vi "Unflatten.vi"(7 "Release Lock":bool=TRUE, 8 "error in (no error)":errorcluster, 9 "Timeout":bool, 10 "DAQ In":T1[](array[typedef]), 11 "CIF_NIChn_FIFO_DAQ in":refnum<class "CIF_NIChn_FIFO_DAQ_DVR.lvclass">) -> (0 "error out":errorcluster, 1 "Header":T2, 2 "DAQ Out":T1[](array[typedef]), 3 "CIF_NIChn_FIFO_DAQ out":refnum<class "CIF_NIChn_FIFO_DAQ_DVR.lvclass">)   [LabVIEW 2021, in "CIF_NIChn_FIFO_DAQ_DVR.lvclass"]
uses:
  CIF_NIChn_FIFO_DAQ_DVR.lvclass
  D:/dev/Packages/Channel_Manager/src/CIFChannels/CIFChannels.lvclass
  D:/dev/Packages/Channel_Manager/src/CIF_NIChn/FIFO_U8/CIF_NIChn_Fifo_U8.lvclass
  ChannelCommon/typedef/FIFO Header.ctl
  ChannelCommon/typedef/Datatype Waveform.ctl
  CIFChannels/CIFChannels.lvclass/CIFChannels.ctl
  FIFO_U8/CIF_NIChn_Fifo_U8.lvclass/CIF_NIChn_Fifo_U8.ctl
  CIF_NIChn_FIFO_DAQ_DVR.lvclass/CIF_NIChn_FIFO_DAQ_DVR.ctl
  <vilib>/CIF Foundation/CIF Utilities/Statistics/I64/Stats_I64_CIF_U.lvclass/Stats_I64_CIF_U.ctl
  4ab41953-a001-49d2-beab-55370b6c3c42.vi
  7cd889b7-face-4678-a9e3-2692853b6930.vi
  CIFChannels/Accessors/Write FIFO Header.vi
  CIFChannels/Accessors/Write FIFO Timeout.vi
  FIFO_U8/Accessors/Read Payload.vi
  ChannelCommon/Utilities/Unflatten Header.vi
  ChannelCommon/Utilities/Add Error.vi
  <vilib>/CIF Foundation/CIF Utilities/DataTypes/Unflatten U64.vi
  <vilib>/CIF Foundation/CIF Utilities/Time/System Time/Get System Time.vi
  <vilib>/CIF Foundation/CIF Utilities/Statistics/I64/X1 minus X0.vi
  <vilib>/CIF Foundation/CIF Utilities/DataTypes/Unflatten I64.vi
  <vilib>/CIF Foundation/CIF Utilities/Errors/Append Error Location.vi
  <vilib>/CIF Foundation/CIF Utilities/Time/System Time/LabVIEW Time to TAI Time.vi
  <vilib>/CIF Foundation/CIF Utilities/Statistics/I64/X1 minus X0.vi/dfabcf33-0dbc-4041-80a5-3dc0c86d2989.vi
  <vilib>/CIF Foundation/CIF Utilities/Statistics/I64/X1 minus X0.vi/dfabcf33-0dbc-4041-80a5-3dc0c86d2989.vi/9eb60a9a-770f-4d2d-8b3f-8465c267ecc9.vi
  ChannelCommon/ChannelCommon.lvlib
  CIFChannels/CIFChannels.lvclass
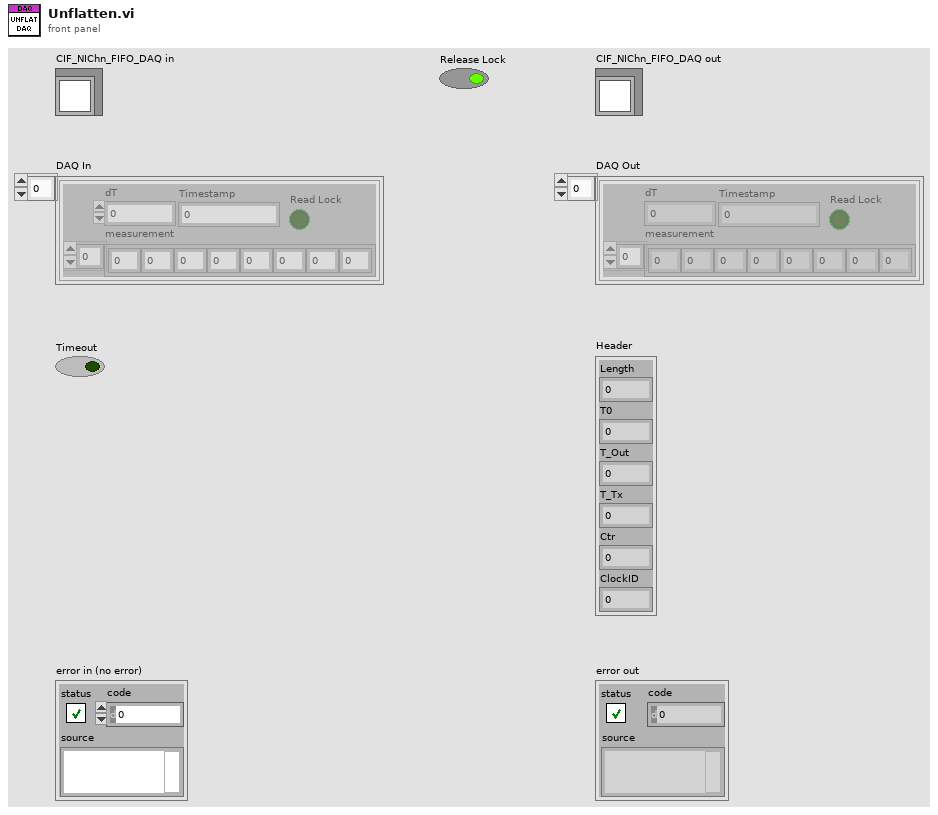
[diagram p1: front panel]
types:
  T1 = typedef "ChannelCommon.lvlib/Datatype Waveform.ctl" = cluster{"measurement":dbl[], "dT":dbl, "Timestamp":i64, "Read Lock":bool}
  T2 = typedef "ChannelCommon.lvlib/FIFO Header.ctl" = cluster{"Length":u64, "T0":i64, "T_Out":i64, "T_Tx":i64, "Ctr":u64, "ClockID":u8}
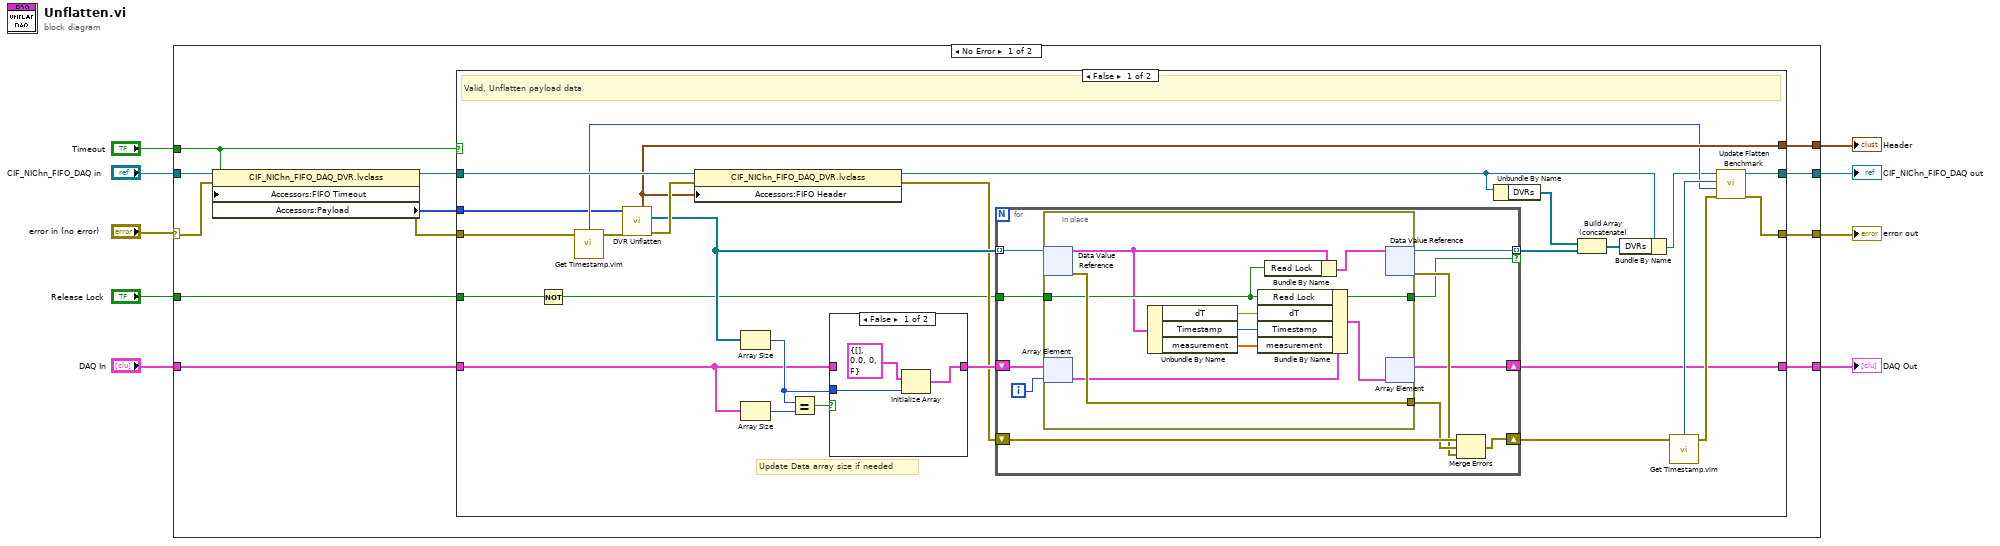
[diagram p0: block diagram]
diagram:
  n1 = case shown="No Error" "error in (no error)" {
    selector: "error in (no error)" -> [w16 w78]
    tunnel: [w19 w78] -> w2
    tunnel: [w20 w77] -> w3
    tunnel: "CIF_NIChn_FIFO_DAQ in" -> [w15 w77]
    tunnel: [w21 _] -> w4
    tunnel: "Timeout" -> [w14 _]
    tunnel: "DAQ In" -> [w13 w76]
    tunnel: [w12 w76] -> w5
    tunnel: "Release Lock" -> [w11 _]
    frame No Error {
      n2 = property class="CIF_NIChn_FIFO_DAQ_DVR.lvclass"(reference=w15, error in=w16, "Accessors:FIFO Timeout"=w14) -> (reference out=w18:refnum<class "CIF_NIChn_FIFO_DAQ_DVR.lvclass">, error out=w17:errorcluster, "Accessors:Payload"=w10:u8[])
      n3 = case shown="False" w14 {
        tunnel: w17 -> [w34 w74]
        tunnel: w18 -> [w47 w75]
        tunnel: [w46 _] -> w21
        tunnel: [w28 w75] -> w20
        tunnel: [w26 w74] -> w19
        tunnel: w13 -> [w30 w73]
        tunnel: [w29 w73] -> w12
        tunnel: w11 -> [w25 _]
        tunnel: w10 -> [w23 _]
        frame False {
          # "Update Data array size if needed"
          # "Valid, Unflatten payload data"
          n4 = Not(x=w25) -> (.not. x?=w24:bool)
          n5 = call "Get Timestamp.vim"("Anything in"=w34) -> ("Time (ns)"=w44:i64, "Anything out"=w33:errorcluster)  [unwired: 2 in]
          n6 = call "DVR Unflatten.vi"("error in (no error)"=w33, "Flatten Data in"=w23) -> ("error out"=w48:errorcluster, "DVRs Out"=w32:refnum<data-value>[], "Header out"=w46:T2)  [unwired: 6 in, 1 out]
          n7 = property class="CIF_NIChn_FIFO_DAQ_DVR.lvclass"(reference=w47, error in=w48, "Accessors:FIFO Header"=w46) -> (reference out=w22:refnum<class "CIF_NIChn_FIFO_DAQ_DVR.lvclass">, error out=w31:errorcluster)
          n8 = Array Size(array=w32) -> (size(s)=w38:i32)
          n9 = Array Size(array=w30) -> (size(s)=w36:i32)
          n10 = Equal?(x=w38, y=w36) -> (x = y?=w35:bool)
          n11 = case shown="False" w35 {
            tunnel: w30 -> [_ w52]
            tunnel: [w49 w52] -> w37
            tunnel: w38 -> [w51 _]
            frame False {
              n12 = Initialize Array(T1 {"measurement"=[], "dT"=0.0, "Timestamp"=0, "Read Lock"=FALSE} ("Waveform Datatype"), w51) -> (w49:T1[])
            }
            frame True {
            }
          }
          n13 = for {
            tunnel: w32 -> [w63] mode=indexing
            shift-right: [w59] -> w39
            shift-left: w31 -> [w62]
            shift-right: [w54] -> w29
            shift-left: w37 -> [w55]
            tunnel: w24 -> [w58]
            tunnel: [w57] -> w42 mode=indexing if=w56
            i -> [w53]
            n14 = in-place {
              in-place-border: [w72] -> w61
              in-place-border: w58 -> [w70]
              in-place-border: [w70] -> w56
              n15 = in-place-dvr #1(w63) -> (w64:T1, w72:errorcluster)
              n16 = in-place-array #2(w55, w53) -> (w66:T1)
              n17 = Unbundle By Name(w64) -> ("dT"=w67:dbl, "Timestamp"=w68:i64, "measurement"=w69:dbl[])
              n18 = Bundle By Name(cluster=w66, "Read Lock"=w70, "dT"=w67, "Timestamp"=w68, "measurement"=w69) -> (w65:T1)
              n19 = Bundle By Name(cluster=w64, "Read Lock"=w70) -> (w71:T1)
              n20 = in-place-dvr #1(w71) -> (w57:refnum<data-value>, w60:errorcluster)
              n21 = in-place-array #2(w65) -> (w54:T1[])  [unwired: 1 out]
            }
            n22 = Merge Errors(w62, w61, w60) -> (w59:errorcluster)
          }
          n23 = Unbundle By Name(w22) -> ("DVRs"=w41:refnum<data-value>[])
          n24 = Build Array (concatenate)(w41, w42) -> (w40:refnum<data-value>[])
          n25 = Bundle By Name(cluster=w22, "DVRs"=w40) -> (w27:refnum<class "CIF_NIChn_FIFO_DAQ_DVR.lvclass">)
          n26 = call "Get Timestamp.vim"("Anything in"=w39) -> ("Time (ns)"=w45:i64, "Anything out"=w43:errorcluster)  [unwired: 2 in]
          n27 = call "Update Flatten Benchmark.vi"("error in (no error)"=w43, "X0"=w44, "X1"=w45, "CIFChannels in"=w27) -> ("error out"=w26:errorcluster, "CIFChannels out"=w28:refnum<class "CIF_NIChn_FIFO_DAQ_DVR.lvclass">)  [unwired: 6 in]
        }
        frame True {
          # "Timeout"
        }
      }
    }
    frame Error {
    }
  }
  "error out" <- w2
  "CIF_NIChn_FIFO_DAQ out" <- w3
  "Header" <- w4
  "DAQ Out" <- w5
